vi "AddSubParsers.vi"(8 "error in (no error)":errorcluster, 10 "SubParserConfig":refnum<class "SubParserConfig.lvclass">, 11 "ArgumentParser in":refnum<class "ArgumentParser.lvclass">) -> (0 "error out":errorcluster, 3 "ArgumentParser out":refnum<class "ArgumentParser.lvclass">)   [LabVIEW 2022 SP3, in "ArgumentParser.lvlib" / "ArgumentParser.lvclass"]
uses:
  ArgumentParser.lvclass
  SubParserConfig/SubParserConfig.lvclass
  SubParserConfig/SubParserConfig.lvclass/SubParserConfig.ctl
  ArgumentParser.lvclass/ArgumentParser.ctl
  SubParserConfig/Read Title.vi
  SubParserConfig/Read Description.vi
  SubParserConfig/Read Program.vi
  SubParserConfig/Read Action.vi
  SubParserConfig/Read Destination.vi
  SubParserConfig/Read Required.vi
  SubParserConfig/Read Help.vi
  SubParserConfig/Read Metavar.vi
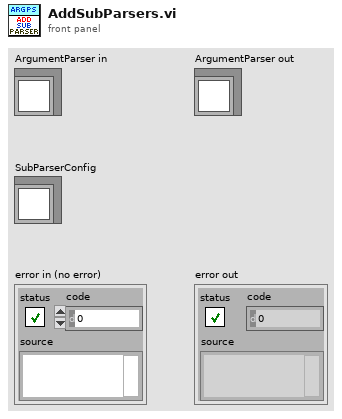
[diagram p1: front panel]
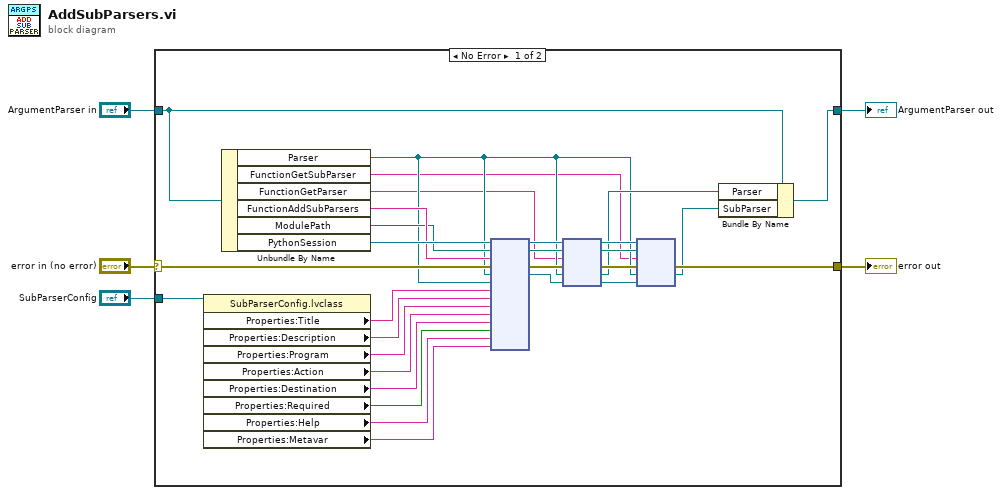
[diagram p0: block diagram]
diagram:
  n1 = case shown="No Error" "error in (no error)" {
    selector: "error in (no error)" -> [w33 w35]
    tunnel: [w15 w35] -> w4
    tunnel: [w23 w34] -> w3
    tunnel: "ArgumentParser in" -> [w22 w34]
    tunnel: "SubParserConfig" -> [w30 _]
    frame No Error {
      n2 = property class="SubParserConfig.lvclass"(reference=w30) -> ("Properties:Title"=w29:string, "Properties:Description"=w28:string, "Properties:Program"=w27:string, "Properties:Action"=w26:string, "Properties:Destination"=w25:string, "Properties:Required"=w24:bool, "Properties:Help"=w21:string, "Properties:Metavar"=w20:string)  [unwired: 1 in, 2 out]
      n3 = Unbundle By Name(w22) -> ("Parser"=w8:refnum<k38>, "FunctionGetSubParser"=w6:string, "FunctionGetParser"=w7:string, "FunctionAddSubParsers"=w31:string, "ModulePath"=w18:path, "PythonSession"=w32:refnum<k35>)
      n4 = node(w32, w18, w31, w33, w8, w8, w29, w28, w27, w26, w25, w24, w21, w20) -> (w19:refnum<k35>, w17:errorcluster, w12:refnum<k38>)  [unwired: 9 in, 2 out]
      n5 = node(w19, w18, w7, w17, w8, w12) -> (w14:refnum<k35>, w13:path, w16:errorcluster, w10:refnum<k38>, w11:refnum<k38>)  [unwired: 1 out]
      n6 = node(w14, w13, w6, w16, w8, w11) -> (w15:errorcluster, w9:refnum<k38>)  [unwired: 1 in, 3 out]
      n7 = Bundle By Name(cluster=w22, "Parser"=w10, "SubParser"=w9) -> (w23:refnum<class "ArgumentParser.lvclass">)
    }
    frame Error {
    }
  }
  "error out" <- w4
  "ArgumentParser out" <- w3
